vi "DC Attenuation Configuration.vi"(6 "Write? (f)":bool, 7 "Connection Refnum":T2, 8 "error in (no error)":errorcluster, 9 "Configuration (\"\")":string, 11 "Template Keys (empty)":T1) -> (0 "error out":errorcluster, 1 "Configuration":string, 3 "Template Keys":T1, 5 "Connection Refnum":T2)   [LabVIEW 2011]
uses:
  Summitek EXT/ODBC/SQL Controls/Connection Refnum.ctl
  ITK EXT/utils/keyedarr.llb/Keyed Array.ctl
  ITK EXT/utils/strutil.llb/Case Matching.ctl
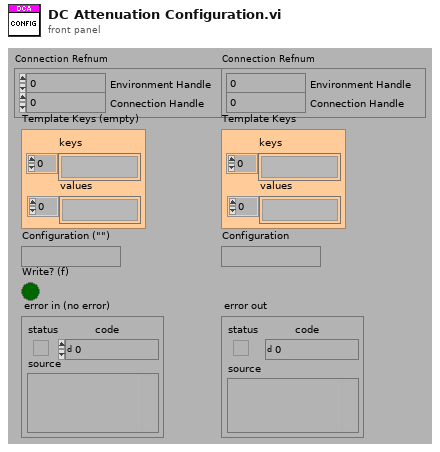
[diagram p1: front panel]
types:
  T1 = typedef "Keyed Array.ctl" = cluster{"keys":string[], "values":string[]}
  T2 = typedef "Connection Refnum.ctl" = cluster{"Environment Handle":i32, "Connection Handle":i32}
  T3 = typedef "Case Matching.ctl" = enum16{"a != A", "a == A", "system"}
  T4 = typedef "DCA Test Parameters.ctl" = cluster{"Stimulus":T5, "Measurement":T6, "Limits":T9[], "Normalization":T14}
  T5 = typedef "DCA Stimulus Parameters.ctl" = cluster{"Use Instrument":bool, "Normalize":bool, "Blank Screen":bool, "Measurement Type":enum16{"Voltage DC", "Voltage DC Ratio", "Voltage AC", "Current DC", "Current AC", "Resistance", "Fresistance", "Frequency", "Period", "Continuity", "Diode"}, "Range":enum16{"Auto", "Minimum", "Maximum", "100", "1,000", "10,000", "100,000", "1,000,000", "10,000,000", "100,000,000"}, "Resolution":enum16{"Auto", "4 1/2", "5 1/2", "6 1/2"}}
  T6 = typedef "DCA Measurement Cluster.ctl" = cluster{"Topology":T7, "Lock Topology":bool, "ATTN Calc":T8, "Zo":dbl}
  T7 = typedef "DCA Topology.ctl" = enum32{"PI-Network", "T-Network"}
  T8 = typedef "DCA Attenuation Calculation.ctl" = enum32{"Power", "Voltage"}
  T9 = typedef "DCA Limit.ctl" = cluster{"Parameter":T10, "Comparison":T11, "Operation":T12, "Value":dbl, "Referential Limit":T13}
  T10 = typedef "DCA Limit Quantity.ctl" = enum16{"Attenuation", "Zin", "Zout", "R1", "R2", "R3", "Rab", "Rac", "Rbc"}
  T11 = typedef "DCA Limit Comparison.ctl" = enum16{">", ">=", "<", "<="}
  T12 = typedef "DCA Limit Operation.ctl" = enum16{"+", "-"}
  T13 = typedef "Test Referential Limit.ctl" = cluster{"Ref Limit":bool, "Ref Type":enum16{"Current", "Specify"}, "Model":string, "Serial":string, "Run Type":enum16{"Most Recent", "Run #", "Match Field"}, "Run":i32, "Field":string, "Field Value":string}
  T14 = typedef "DCA Calibration State.ctl" = cluster{"Normalized?":bool, "Rab Value":dbl, "Rac Value":dbl, "Rbc Value":dbl}
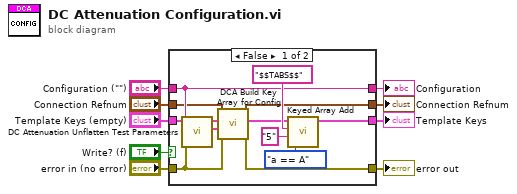
[diagram p0: block diagram]
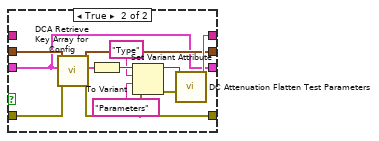
[diagram p2: hidden frame]
diagram:
  n1 = case shown="False" "Write? (f)" {
    tunnel: "error in (no error)" -> [w10 w27]
    tunnel: [w14 w22] -> w8
    tunnel: "Template Keys (empty)" -> [w12 w22]
    tunnel: "Configuration (\"\")" -> [w18 _]
    tunnel: [w13 w26] -> w5
    tunnel: [w18 w28] -> w4
    tunnel: "Connection Refnum" -> [w17 w25]
    tunnel: [w16 w24] -> w1
    frame False {
      n2 = call "DC Attenuation Unflatten Test Parameters.vi"("error in (no error)"=w10, "Parameter String"=w18) -> ("DC Attenuation Test Parameters"=w11:T4)  [unwired: 9 out]
      n3 = call "DCA Build Key Array for Config.vi"("error in (no error)"=w10, "DC Attenuation Test Parameters"=w11, "Key Array In"=w12, "Connection Refnum"=w17) -> ("error out"=w13:errorcluster, "Key Array Out"=w15:T1, "Connection Refnum"=w16:T2)  [unwired: 5 out]
      n4 = call "Keyed Array Add.vi"("case matching (sensitive)"=Case_Matching."a == A", "value"="5", "key"="$$TABS$$", "array in"=w15) -> ("array out"=w14:T1)  [unwired: 3 out]
    }
    frame True {
      n5 = call "DCA Retrieve Key Array for Config.vi"("error in (no error)"=w27, "Key Array In"=w22, "Connection Refnum"=w25) -> ("error out"=w26:errorcluster, "DCA Test Parameters"=w23:T4, "Connection Refnum"=w24:T2)  [unwired: 1 in, 5 out]
      n6 = To Variant(anything=w23) -> (Variant=w33:variant)
      n7 = Set Variant Attribute(Variant=w33, name="Type", value="Parameters" ("name"), error in=w26) -> (Variant out=w29:variant, error out=w32:errorcluster)  [unwired: 1 out]
      n8 = call "DC Attenuation Flatten Test Parameters.vi"("error in (no error)"=w32, "Parameter Variant"=w29) -> ("Parameter String"=w28:string)  [unwired: 9 out]
    }
  }
  "error out" <- w5
  "Connection Refnum" <- w1
  "Template Keys" <- w8
  "Configuration" <- w4
